vi "check_blank_eid.vi"(8 "error in (no error)":errorcluster, 10 "eid in":string, 11 "Device In":T1) -> (0 "error out":errorcluster, 2 "Device Out":T1, 3 "eid out":string)   [LabVIEW 2019]
uses:
  <userlib>/Onshape/_SubVI/Cluster.ctl
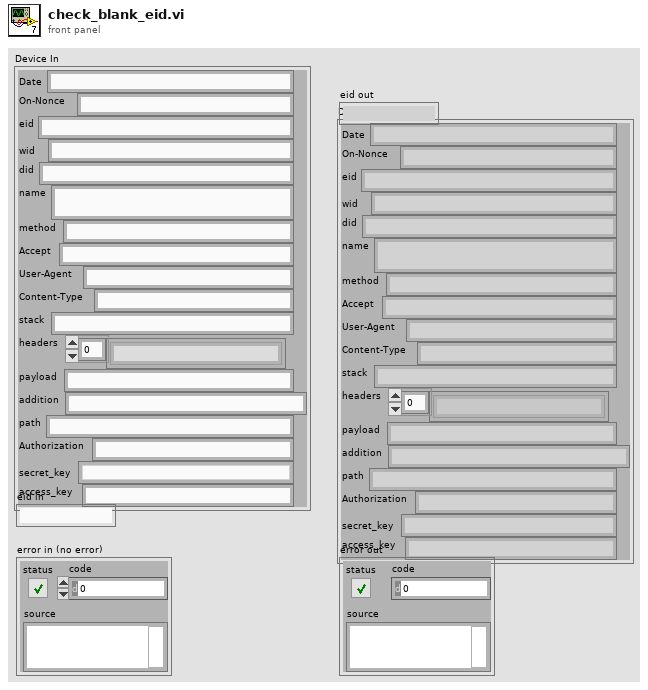
[diagram p1: front panel]
types:
  T1 = typedef "Cluster.ctl" = cluster{"Date":string, "On-Nonce":string, "eid":string, "wid":string, "did":string, "name":string, "method":string, "Accept":string, "User-Agent":string, "Content-Type":string, "stack":string, "headers":string[], "payload":string, "addition":string, "path":string, "Authorization":string, "secret_key":string, "access_key":string}
  T2 = cluster{"id":string, "elementType":string, "name":string}[]
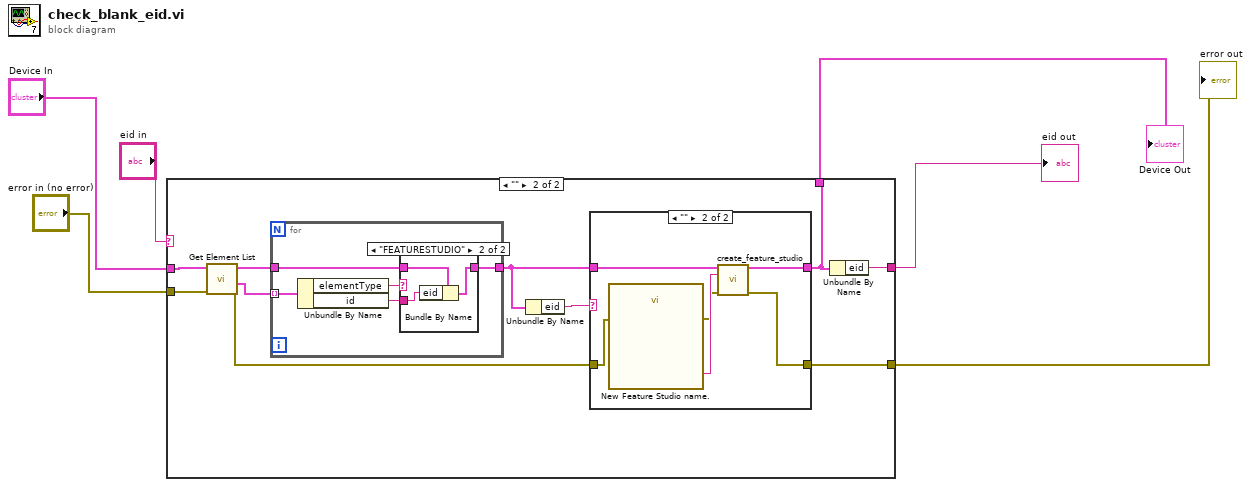
[diagram p0: block diagram]
diagram:
  n1 = case shown="\"\"" "eid in" {
    selector: "eid in" -> [w9 _]
    tunnel: "Device In" -> [w7 w19]
    tunnel: [w9 w13] -> w2
    tunnel: "error in (no error)" -> [w8 w16]
    tunnel: [w8 w12] -> w4
    tunnel: [w7 w10] -> w6
    frame Default {
    }
    frame "" {
      n2 = call <userlib>:"Get Element List.vi"("error in"=w16, "Device In"=w19) -> ("error out"=w14:errorcluster, "value"=w18:T2, "Device Out"=w17:T1)  [unwired: 6 in, 1 out]
      n3 = for {
        tunnel: w18 -> [w31] mode=indexing
        tunnel: w17 -> [w28]
        tunnel: [w29] -> w11
        n4 = Unbundle By Name(w31) -> ("elementType"=w32:string, "id"=w30:string)
        n5 = case shown="\"FEATURESTUDIO\"" w32 {
          tunnel: w28 -> [w33 w35]
          tunnel: w30 -> [_ w36]
          tunnel: [w33 w34] -> w29
          frame Default {
          }
          frame "FEATURESTUDIO" {
            n6 = Bundle By Name(cluster=w35, "eid"=w36) -> (w34:T1)
          }
        }
      }
      n7 = Unbundle By Name(w11) -> ("eid"=w15:string)
      n8 = case shown="\"\"" w15 {
        tunnel: w11 -> [w21 w27]
        tunnel: [w21 w25] -> w10
        tunnel: w14 -> [w20 w24]
        tunnel: [w20 w22] -> w12
        frame Default {
        }
        frame "" {
          n9 = call "New Feature Studio name."("error in (no error)"=w24) -> ("New Feature Studio Name"=w26:string, "error out"=w23:errorcluster)  [unwired: 16 in, 1 out]
          n10 = call <userlib>:"create_feature_studio.vi"("Device In"=w27, "New Feature Studio Name"=w26, "error in"=w23) -> ("Device Out"=w25:T1, "error out"=w22:errorcluster)  [unwired: 10 in, 1 out]
        }
      }
      n11 = Unbundle By Name(w10) -> ("eid"=w13:string)
    }
  }
  "Device Out" <- w6
  "error out" <- w4
  "eid out" <- w2
